vi "low_pass_filter_2rd.vi"(7 "Input":dbl format="%.2f", 13 "Corner period":dbl(slide)=10.237739663395852 scale=1.0..1000.0) -> (8 "Output":dbl format="%.2f")   [LabVIEW 2016]
doc: "Use this VI to filter a signal using 2nd order low pass filter. The difference equation is \n[y(j)-2*y(j-1)+y(j-2)] + sqrt(2)*b*[y(j)-y(j-1)] + (b^2)*y(j) = (b^2)*x(j).\n\nInputs:\nInput,\nCorner period.\nOutputs:\nOutput.\n\nMuhannad Alghamdi\nCSUSB Physics 350"
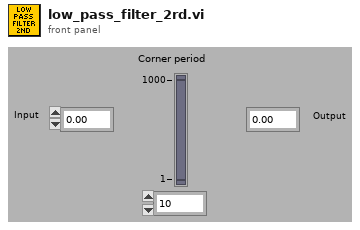
[diagram p1: front panel]
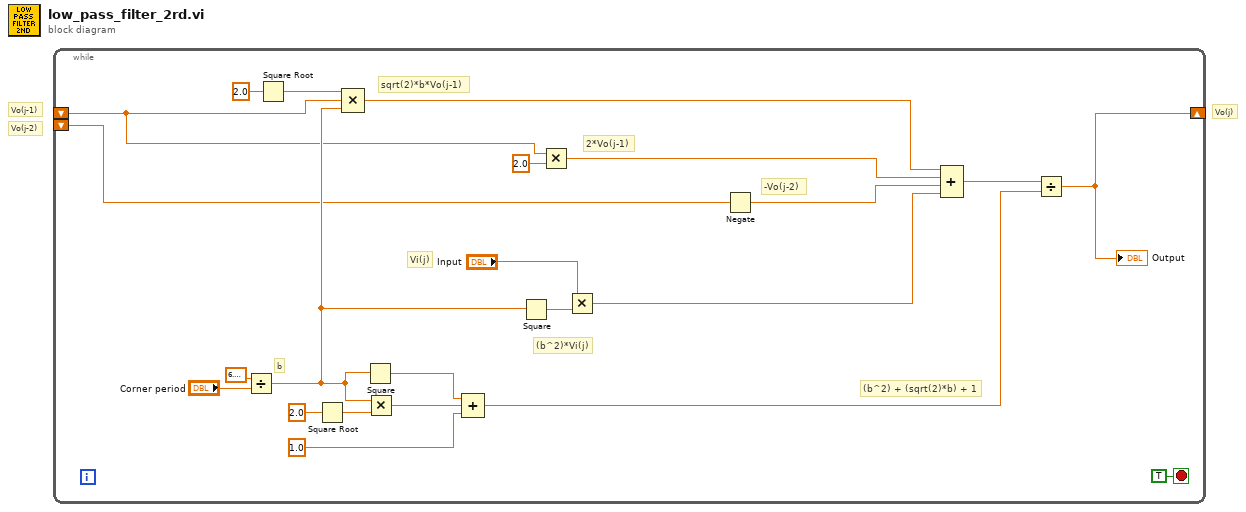
[diagram p0: block diagram]
diagram:
  # "Vo(j-1)"
  # "Vo(j-2)"
  # "Vo(j)"
  n1 = while {
    shift-left: _ -> [w4]
    shift-right: [w18] -> _
    shift-left: _ -> [w2]
    stop <- TRUE stop-if-true
    # "-Vo(j-2)"
    # "2*Vo(j-1)"
    # "(b^2)*Vi(j)"
    # "sqrt(2)*b*Vo(j-1)"
    # "Vi(j)"
    # "(b^2) + (sqrt(2)*b) + 1"
    # "b"
    n2 = Divide(x=6.283185307179586, y="Corner period") -> (x/y=w7:dbl)
    n3 = Square Root(x=2.0) -> (sqrt(x)=w8:dbl)
    n4 = Square Root(x=2.0) -> (sqrt(x)=w15:dbl)
    n5 = Compound Arithmetic op=MULTIPLY(w8, w4, w7) -> (w9:dbl)
    n6 = Square(x=w7) -> (x^2=w14:dbl)
    n7 = Multiply(x=w7, y=w15) -> (x*y=w13:dbl)
    n8 = Compound Arithmetic op=ADD(w14, w13, 1.0 ("value")) -> (w17:dbl)
    n9 = Square(x=w7) -> (x^2=w11:dbl)
    n10 = Multiply(x=w4, y=2.0) -> (x*y=w3:dbl)
    n11 = Multiply(x="Input", y=w11) -> (x*y=w6:dbl)
    n12 = Negate(x=w2) -> (-x=w1:dbl)
    n13 = Compound Arithmetic op=ADD(w9, w3, w1, w6) -> (w19:dbl)
    n14 = Divide(x=w19, y=w17) -> (x/y=w18:dbl)
    "Output" <- w18
  }
